vi "Get Legend Axis.vi"(8 "error in (no error)":errorcluster, 11 "3D Contour in":refnum<class "3D Contour.lvclass">) -> (0 "error out":errorcluster, 1 "Active Axis":enum16{"X-axis", "Y-axis", "Z-axis"}(ring)=enum."Z-axis", 3 "3D Contour out":refnum<class "3D Contour.lvclass">)   [LabVIEW 2020, in "3D Contour.lvclass"]
uses:
  <vilib>/Math Plots/3D Math Plots/3D Contour/3D Contour/3D Contour.lvclass
  e:/builds/penguin/labview/branches/2020/dev/dist/vi.lib/Math Plots/3D Math Plots/3D Plot/3D Plot/3D Plot.lvclass
  <vilib>/Math Plots/3D Math Plots/3D Contour/3D Contour/3D Contour.lvclass/3D Contour.ctl
  <vilib>/Math Plots/3D Math Plots/3D Plot/3D Plot/3D Plot.lvclass
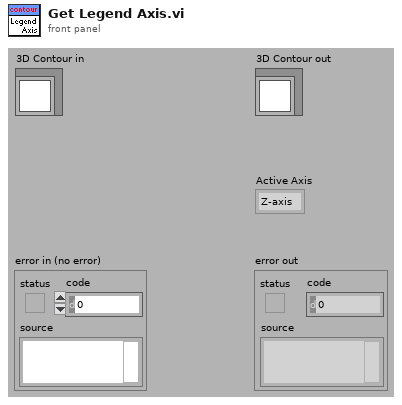
[diagram p1: front panel]
types:
  T1 = typedef "3D Contour.lvclass/3D Contour Property Array.ctl" = T2[]
  T2 = typedef "3D Contour.lvclass/3D Contour Property.ctl" = cluster{"General Property":cluster{"Plot Name":string, "Coordinate System":enum16{"Cartesian", "Cylindrical", "Spherical"}, "Opacity":sgl}, "Projection Property":cluster{"Draw XY":bool, "Draw YZ":bool, "Draw XZ":bool}, "Plot Property":cluster{"Line Style":T3, "Line Width":sgl, "Line Color":u32, "Antialiasing":bool, "Color Ramp Cluster":T4}, "Contour Property":cluster{"Contour Type":enum16{"Contour", "Contour with surface"}, "Axis Basis":enum16{"X-Axis", "Y-Axis", "Z-Axis"}, "Level List":sgl[], "Level Mode":enum16{"Levels", "Interval", "Level List"}, "Levels":u16, "Interval":sgl}}
  T3 = typedef "3D Plot.lvclass/Line Type.ctl" = enum16{"None", "Solid", "Dash", "Dot", "Dash Dot"}
  T4 = typedef "3D Plot.lvclass/Color Ramp Cluster.ctl" = cluster{"Color Ramp Style":enum16{"None", "Shaded", "Color spectrum", "Grey scale", "Custom"}, "Color Ramp Array":u32[], "Color Ramp Index":i32[], "Interpolate?":bool, "Logarithm?":bool}
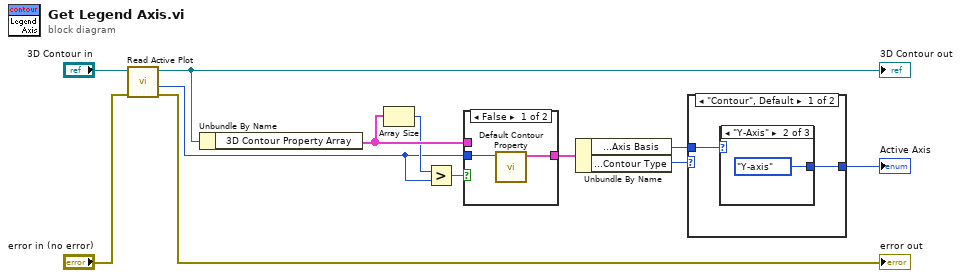
[diagram p0: block diagram]
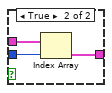
[diagram p2: hidden frame]
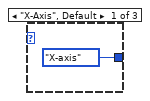
[diagram p3: hidden frame]
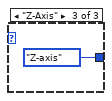
[diagram p4: hidden frame]
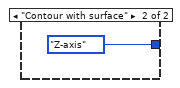
[diagram p5: hidden frame]
diagram:
  n1 = call <vilib>:"Read Active Plot.vi"("error in (no error)"="error in (no error)", "3D Plot.lvclass in"="3D Contour in") -> ("error out"=→"error out":errorcluster, "Active Plot"=w2:i32, "3D Plot.lvclass out"=w9:refnum<class "3D Contour.lvclass">)  [unwired: 7 out]
  "3D Contour out" <- w9
  n2 = Unbundle By Name(w9) -> ("3D Contour Property Array"=w4:T1)
  n3 = Array Size(array=w4) -> (size(s)=w3:i32)
  n4 = Greater?(x=w3, y=w2) -> (0:w1:bool)
  n5 = case shown="False" w1 {
    tunnel: w2 -> [w14 w17]
    tunnel: [w13 w16] -> w12
    tunnel: w4 -> [_ w15]
    frame False {
      n6 = call <vilib>:"Default Contour Property.vi"("Plot ID"=w14) -> ("Default Property"=w13:T2)  [unwired: 10 out]
    }
    frame True {
      n7 = Index Array(array=w15, index=w17) -> (element=w16:T2)
    }
  }
  n8 = Unbundle By Name(w12) -> ("Contour Property.Axis Basis"=w11:enum16{"X-Axis", "Y-Axis", "Z-Axis"}, "Contour Property.Contour Type"=w5:enum16{"Contour", "Contour with surface"})
  n9 = case shown="\"Contour\", Default" w5 {
    tunnel: w11 -> [w19 _]
    tunnel: [w18 enum16{"X-axis", "Y-axis", "Z-axis"}."Z-axis" ("Active Axis")] -> w6
    frame "Contour", Default {
      n10 = case shown="\"Y-Axis\"" w19 {
        tunnel: [enum16{"X-axis", "Y-axis", "Z-axis"}."X-axis" ("Active Axis") enum16{"X-axis", "Y-axis", "Z-axis"}."Y-axis" ("Active Axis") enum16{"X-axis", "Y-axis", "Z-axis"}."Z-axis" ("Active Axis")] -> w18
        frame "X-Axis", Default {
        }
        frame "Y-Axis" {
        }
        frame "Z-Axis" {
        }
      }
    }
    frame "Contour with surface" {
    }
  }
  "Active Axis" <- w6
